vi "NR Select and Initiate Measurements.vi"(0 "Instrument Handle In":refnum<k21>, 1 "Selector String":string, 2 "Result Name":string, 5 "Measurements":T1(array[ring]), 7 "Auto Level Configuration":T2={"Enabled"=FALSE, "Measurement Interval (s)"=0.01} {"Measurement Interval (s)" min=1e-06 max=100.0 format="%.2p"}, 11 "error in (no error)":errorcluster, 12 "Enable All Traces (F)":bool) -> (4 "Instrument Handle Out":refnum<k21>, 6 "Selector String Out":string, 15 "error out":errorcluster)   [LabVIEW 2016, in "RFmxNR.lvlib"]
doc: "Performs actions to initiate acquisition and measurement. \n\nEnables the specified measurement(s) before optionally automatically adjusting the reference level before beginning measurements. Finally, initiates the acquisition and measurement(s)."
uses:
  RFmxNR.lvlib
  Common/SA Auto Level Configuration.ctl
  <vilib>/RFmx/NR/mx/RFmxNR.llb/RFmxNR Select Measurement (Multiple).vi
  Common/Common.lvlib
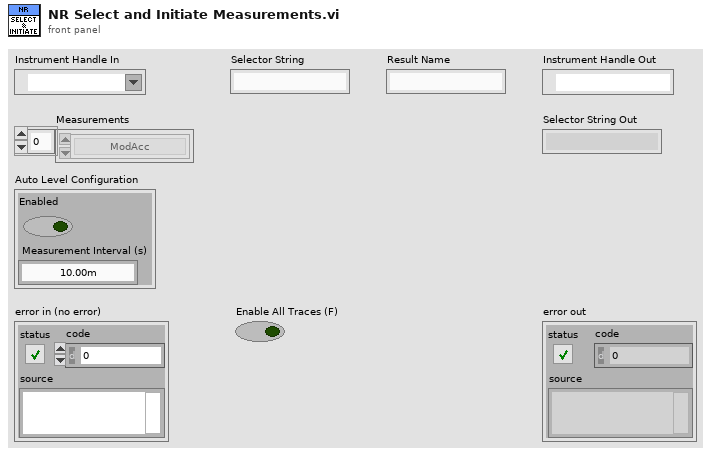
[diagram p1: front panel]
types:
  T1 = enum16{"ModAcc", "SEM", "ACP", "CHP", "OBW", "PVT"}[]
  T2 = typedef "Common.lvlib/SA Auto Level Configuration.ctl" = cluster{"Enabled":bool, "Measurement Interval (s)":dbl}
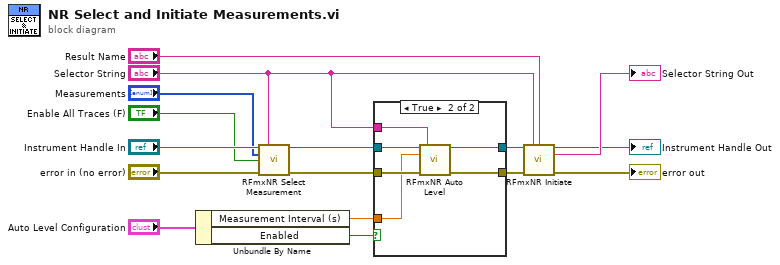
[diagram p0: block diagram]
diagram:
  n1 = Unbundle By Name("Auto Level Configuration") -> ("Measurement Interval (s)"=w3:dbl, "Enabled"=w4:bool)
  n2 = call-poly <vilib>:"RFmxNR Select Measurement.vi"("Instrument Handle In"="Instrument Handle In", "Selector String"="Selector String", "Measurements"="Measurements", "Enable All Traces"="Enable All Traces (F)", "error in (no error)"="error in (no error)") -> ("Instrument Handle Out"=w7:refnum<k21>, "error out"=w13:errorcluster)  [unwired: 9 in]
  n3 = case shown="True" w4 {
    tunnel: w13 -> [w17 w24]
    tunnel: [w17 w23] -> w8
    tunnel: w7 -> [w18 w22]
    tunnel: [w18 w21] -> w6
    tunnel: w3 -> [_ w20]
    tunnel: "Selector String" -> [_ w19]
    frame False {
    }
    frame True {
      n4 = call <vilib>:"RFmxNR Auto Level.vi"("Instrument Handle In"=w22, "Selector String"=w19, "Measurement Interval (s)"=w20, "error in (no error)"=w24) -> ("Instrument Handle Out"=w21:refnum<k21>, "error out"=w23:errorcluster)  [unwired: 9 in, 1 out]
    }
  }
  n5 = call <vilib>:"RFmxNR Initiate.vi"("Instrument Handle In"=w6, "Selector String"="Selector String", "Result Name"="Result Name", "error in (no error)"=w8) -> ("Instrument Handle Out"=→"Instrument Handle Out":refnum<k21>, "Selector String Out"=→"Selector String Out":string, "error out"=→"error out":errorcluster)  [unwired: 9 in]
